vi "List All SystemLink Feeds.vi"(0 "SystemLink repo in":T1, 11 "error in (no error)":errorcluster) -> (4 "SystemLink repo out":T1, 6 "SystemLink Feed Names":string[](array[string]), 8 "SystemLink Feed IDs":string[](array[string]), 15 "error out":errorcluster)   [LabVIEW 2017, in "SystemLink_Repo_API.lvlib"]
doc: "Lists all the feeds in the SystemLink repository.\n\nOutputs:\nSystemLink Feed Names - a 1D array containing the names of all the feeds in the SystemLink repository.\n\nSystemLink Feed IDs - a 1D array containing the Feed IDs that correspond to the feed names in the SystemLink Feed Names output."
uses:
  SystemLink_Repo_API.lvlib
  _support/systemlink repo.ctl
  <vilib>/httpClient/ClientHandle.ctl
  0e4db4ab-2fe0-46a1-a8ee-8182cf8a8e9d.vi
  <vilib>/JDP Science/JSONtext/Find Multiple Items.vi
  <vilib>/JDP Science/JSONtext/String Subset.vi
  <vilib>/JDP Science/JSONtext/support/Strip Quotes and Unescape.vi
  <vilib>/JDP Science/JSONtext/Parsing/Parse Full Path or Item Name.vi
  <vilib>/JDP Science/JSONtext/Offset/Find Item Locations by Path.vi
  <vilib>/JDP Science/JSONtext/support/Unescape JSON string.vi
  <vilib>/JDP Science/JSONtext/JSON text to Variant.vi
  <vilib>/httpClient/LabVIEWHTTPClient.lvlib
panel:
  out "body":string
  out "headers":string
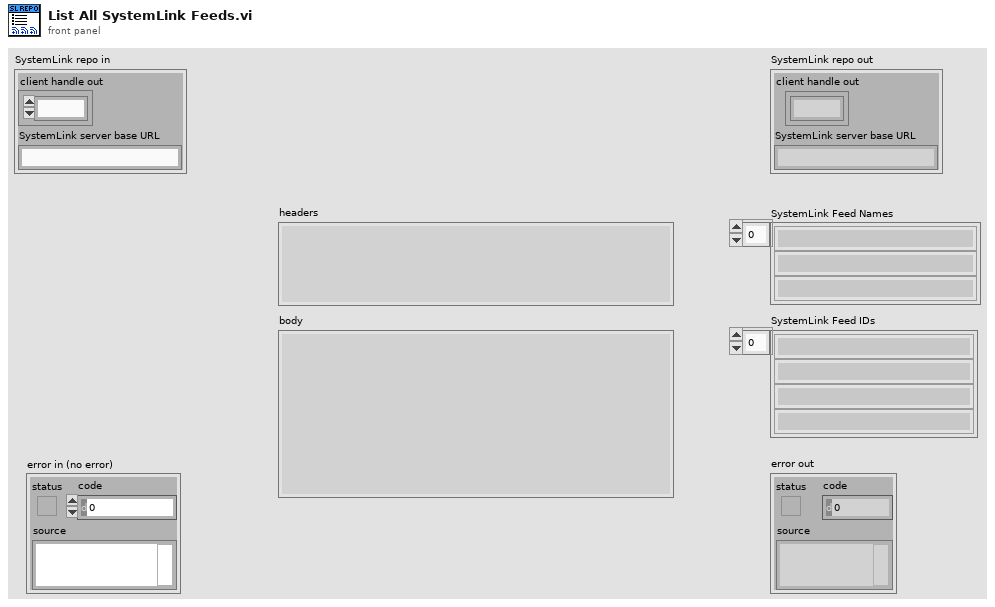
[diagram p1: front panel]
types:
  T1 = typedef "SystemLink_Repo_API.lvlib/systemlink repo.ctl" = cluster{"client handle out":T2, "SystemLink server base URL":string}
  T2 = typedef "LabVIEWHTTPClient.lvlib/ClientHandle.ctl" = refnum<k1>
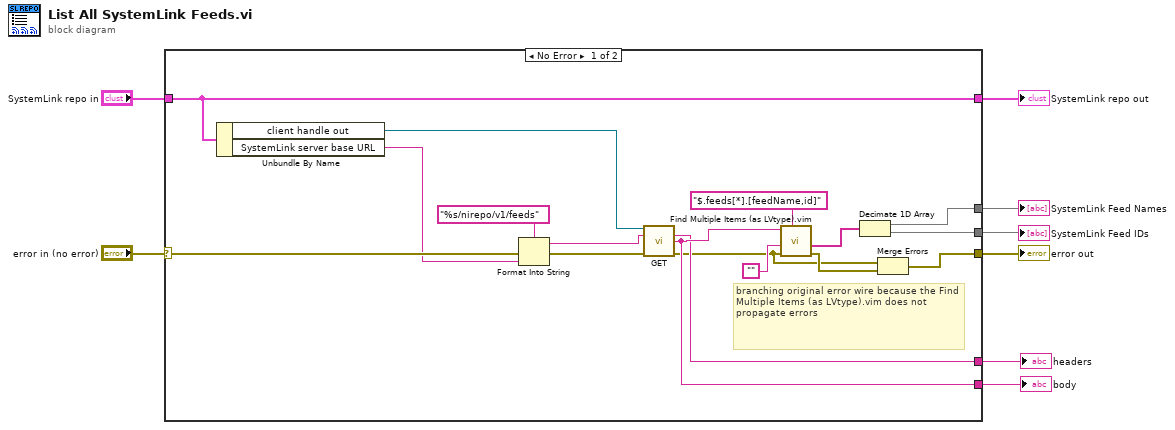
[diagram p0: block diagram]
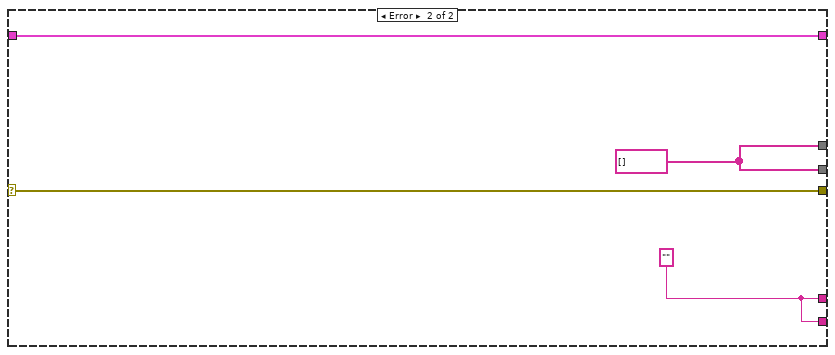
[diagram p2: hidden frame]
diagram:
  n1 = case shown="No Error" "error in (no error)" {
    selector: "error in (no error)" -> [w22 w29]
    tunnel: "SystemLink repo in" -> [w14 w27]
    tunnel: [w11 w29] -> w6
    tunnel: [w13 w26] -> w5
    tunnel: [w16 w28] -> w4
    tunnel: [w15 w28] -> w3
    tunnel: [w14 w27] -> w2
    tunnel: [w12 w26] -> w1
    frame No Error {
      # "branching original error wire because the Find Multiple Items (as LVtype).vim does not propagate errors"
      n2 = Unbundle By Name(w14) -> ("client handle out"=w23:T2, "SystemLink server base URL"=w17:string)
      n3 = Format Into String(format string="%s/nirepo/v1/feeds", error in=w22, w17) -> (resulting string=w24:string, error out=w21:errorcluster)  [unwired: 1 in]
      n4 = call <vilib>:"GET.vi"("client handle"=w23, "url"=w24, "error in (no error)"=w21) -> ("headers"=w15:string, "body"=w16:string, "error out"=w9:errorcluster)  [unwired: 9 in, 1 out]
      n5 = call "Find Multiple Items (as LVtype).vim"("$Path or Item Name"="$.feeds[*].[feedName,id]", "error in (no error)"=w9, "Data Type and Default Value"="", "JSON"=w16) -> ("error out"=w10:errorcluster, "Array of Data"=w18:string[])  [unwired: 4 in, 2 out]
      n6 = Decimate 1D Array(w18) -> (w13:string[], w12:string[])
      n7 = Merge Errors(w9, w10) -> (w11:errorcluster)
    }
    frame Error {
      w28 = "" ("headers")
      w26 = string[] [] ("Array of Data")
    }
  }
  "error out" <- w6
  "SystemLink repo out" <- w2
  "SystemLink Feed Names" <- w5
  "headers" <- w3
  "body" <- w4
  "SystemLink Feed IDs" <- w1
